vi "QRcode.vi"() -> ()   [LabVIEW 2020]
uses:
  <vilib>/vision/Instrument.llb/QR Code Report.ctl
  <vilib>/vision/Instrument.llb/QR Code Model Type.ctl
  <vilib>/vision/Instrument.llb/QR Code Stream Mode Type.ctl
  <vilib>/vision/Instrument.llb/Data Matrix Polarity.ctl
  <vilib>/vision/Instrument.llb/Demodulation Mode.ctl
  <vilib>/vision/Instrument.llb/Cell Sample Size.ctl
  <vilib>/vision/Instrument.llb/Cell Filter Mode.ctl
panel:
  out "Array 2":bool[](array[boolean])
  out "Array":string[](array[string])
  in  "ROT":dbl
  in  "B":dbl
  in  "T":dbl
  out "QR Barcode Report (2D Barcode Reader 1)":T1={"Found?"=FALSE, "Data"="", "Bounding Box"=[], "Errors Corrected"=0, "Dimensions (Rows/Cols)"=0, "Version"=0, "QR Model"=3, "Stream Mode"=0, "Barcode Polarity"=-2, "Mirrored?"=FALSE, "Append Stream Position"=0, "Size of Append Stream"=0, "First EAN-128 ID"=0, "First Alternate Language ID"=0, "Append Stream ID"=0, "Minimum Edge Strength"=30, "Demodulation Mode"=-2, "Cell Sample Size"=-2, "Cell Filter Mode"=-2} {"Append Stream ID" format="%x"; "Cell Filter Mode" items=["Auto-detect"=-2, "Average"=0, "Median"=1, "Central Average"=2, "High Average"=3, "Low Average"=4, "Very High Average"=5, "Very Low Average"=6, "All Filters"=8]; "Cell Sample Size" items=["Auto-detect"=-2, "1x1"=1, "2x2"=2, "3x3"=3, "4x4"=4, "5x5"=5, "6x6"=6, "7x7"=7]; "Demodulation Mode" items=["Auto-detect"=-2, "Histogram"=0, "Local Contrast"=1, "Combination"=2, "All"=3]; "Barcode Polarity" items=["Auto-detect"=-2, "Black on White"=0, "White on Black"=1]; "Stream Mode" items=["Auto-detect", "Numeric", "AlphaNumeric", "Mixed", "Raw Bytes", "UCC/EAN-128 - In Tokens", "UCC/EAN-128 - In Data", "Extended Character Interpretation", "Kanji"]; "QR Model" items=["Auto Detect", "Micro", "Model 1", "Model 2"]; "Version" max=40 step=1}
  in  "Stop (F)":bool
  out "Image Out":T8(plugin-control)
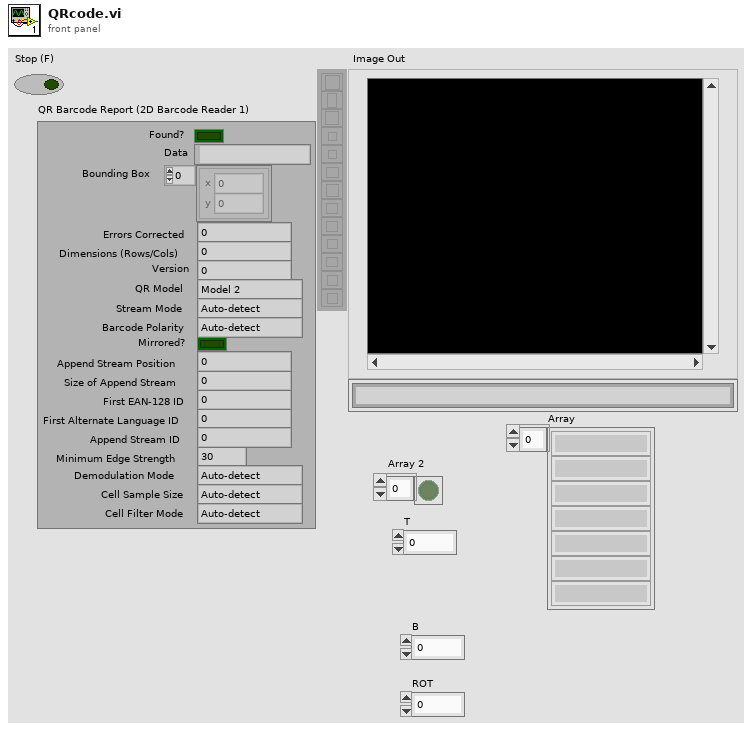
[diagram p1: front panel]
types:
  T1 = typedef "QR Code Report.ctl" = cluster{"Found?":bool, "Data":string, "Bounding Box":cluster{"x":sgl, "y":sgl}[], "Errors Corrected":u32, "Dimensions (Rows/Cols)":u32, "Version":u32, "QR Model":T2, "Stream Mode":T3, "Barcode Polarity":T4, "Mirrored?":bool, "Append Stream Position":u32, "Size of Append Stream":u32, "First EAN-128 ID":i32, "First Alternate Language ID":i32, "Append Stream ID":u32, "Minimum Edge Strength":u32, "Demodulation Mode":T5, "Cell Sample Size":T6, "Cell Filter Mode":T7}
  T2 = typedef "QR Code Model Type.ctl" = i32
  T3 = typedef "QR Code Stream Mode Type.ctl" = i32
  T4 = typedef "Data Matrix Polarity.ctl" = i32
  T5 = typedef "Demodulation Mode.ctl" = i32
  T6 = typedef "Cell Sample Size.ctl" = i32
  T7 = typedef "Cell Filter Mode.ctl" = i32
  T8 = typedef "IMAQ Image.ctl" = refnum<image>
  T9 = typedef "ROI Descriptor" = cluster{"Global Rectangle":i32[], "Contours":cluster{"ID":enum32{"External", "Internal"}, "Type":u32, "Coordinates":i32[]}[]}
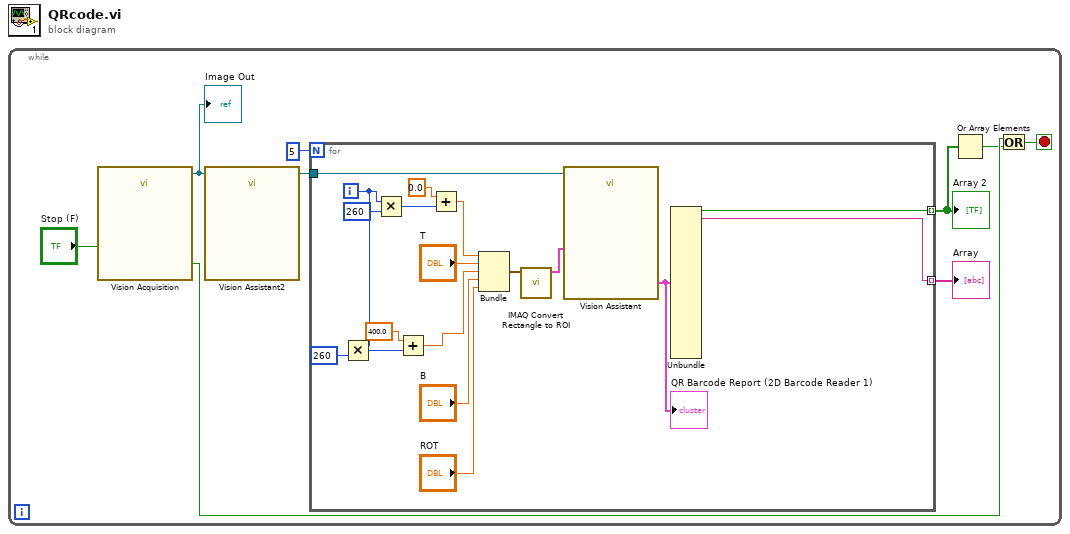
[diagram p0: block diagram]
diagram:
  n1 = while {
    stop <- w2 stop-if-true
    n2 = call "Vision Acquisition"("Stop (F)"="Stop (F)") -> ("Image Out"=w6:T8, "Stopped"=w3:bool)  [unwired: 24 in, 1 out]
    "Image Out" <- w6
    n3 = call "Vision Assistant2"("Image In"=w6) -> ("Image Out"=w5:T8)  [unwired: 25 in, 1 out]
    n4 = for {
      N: 5 -> [_]
      tunnel: w5 -> [w24]
      tunnel: [w22] -> w7 mode=indexing
      tunnel: [w15] -> w4 mode=indexing
      i -> [w10]
      n5 = Multiply(x=w10, y=260) -> (x*y=w12:i32)
      n6 = Multiply(x=w10, y=260) -> (x*y=w21:i32)
      n7 = Add(x=400.0, y=w12) -> (x+y=w11:dbl)
      n8 = Add(x=0.0, y=w21) -> (x+y=w18:dbl)
      n9 = Bundle(w18, "T"="T", w11, "B"="B", "ROT"="ROT") -> (w17:cluster{dbl, "T":dbl, dbl, "B":dbl, "ROT":dbl})  [unwired: 1 in]
      n10 = call "IMAQ Convert Rectangle to ROI"("Rectangle"=w17) -> ("ROI Descriptor"=w16:T9)  [unwired: 8 in, 1 out]
      n11 = call "Vision Assistant"("Image In"=w24, "ROI Descriptor (2D Barcode Reader 1)"=w16) -> ("QR Barcode Report (2D Barcode Reader 1)"=w23:T1)  [unwired: 23 in, 2 out]
      "QR Barcode Report (2D Barcode Reader 1)" <- w23
      n12 = Unbundle(w23) -> ("Found?"=w15:bool, "Data"=w22:string)  [unwired: 17 out]
    }
    "Array" <- w7
    "Array 2" <- w4
    n13 = Or Array Elements(Boolean array=w4) -> (logical OR=w1:bool)
    n14 = Or(x=w3, y=w1) -> (x .or. y?=w2:bool)
  }
